vi "Add Address Map Element.vi"(0 "niInstr AXI4-Lite address space v1 FPGA in":refnum<class "niInstr AXI4-Lite Address Space v1 FPGA.lvclass">, 5 "address map element in":T1) -> (4 "niInstr AXI4-Lite address space v1 FPGA out":refnum<class "niInstr AXI4-Lite Address Space v1 FPGA.lvclass">)   [LabVIEW 2015, in "niInstr AXI4-Lite Address Space v1 FPGA.lvclass"]
uses:
  <instrlib>/_niInstr/CLIP Adapters/v1/FPGA/AXI4-Lite/Address Space/niInstr AXI4-Lite Address Space v1 FPGA.lvclass
  <instrlib>/_niInstr/Instruction Framework/v1/FPGA/Typedefs/Address Map Element.ctl
  <instrlib>/_niInstr/CLIP Adapters/v1/FPGA/AXI4-Lite/Address Space/niInstr AXI4-Lite Address Space v1 FPGA.lvclass/niInstr AXI4-Lite Address Space v1 FPGA.ctl
  <instrlib>/_niInstr/Instruction Framework/v1/FPGA/Typedefs/niInstr Instruction Framework v1 FPGA.lvlib
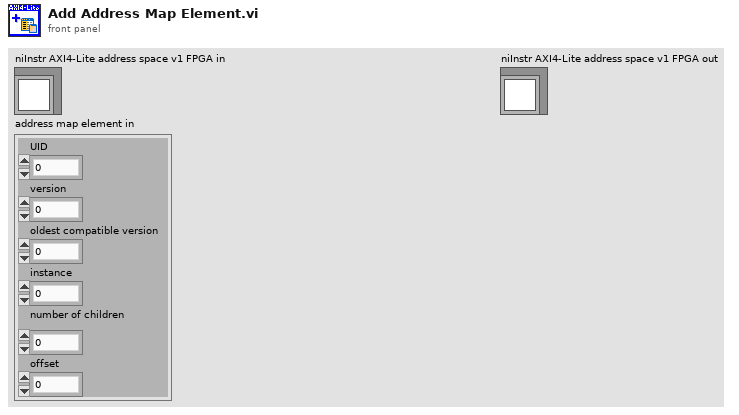
[diagram p1: front panel]
types:
  T1 = typedef "niInstr Instruction Framework v1 FPGA.lvlib/Address Map Element.ctl" = cluster{"UID":u16, "version":u16, "oldest compatible version":u16, "instance":u8, "number of children":u8, "offset":u32}
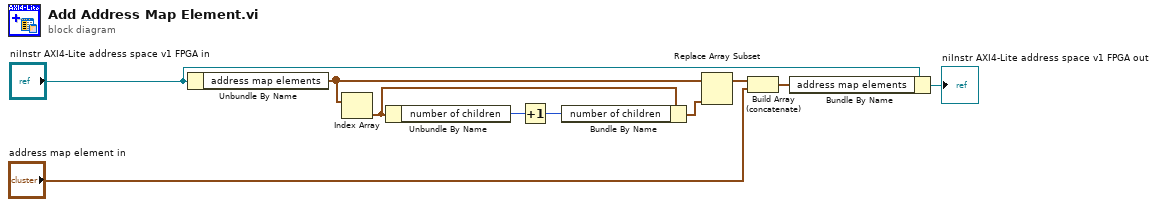
[diagram p0: block diagram]
diagram:
  n1 = Unbundle By Name("niInstr AXI4-Lite address space v1 FPGA in") -> ("address map elements"=w5:T1[])
  n2 = Index Array(array=w5) -> (element=w7:T1)  [unwired: 1 in]
  n3 = Unbundle By Name(w7) -> ("number of children"=w6:u8)
  n4 = Increment(x=w6) -> (x+1=w1:u8)
  n5 = Bundle By Name(cluster=w7, "number of children"=w1) -> (w4:T1)
  n6 = Replace Array Subset(array=w5, new element=w4) -> (w3:T1[])  [unwired: 1 in]
  n7 = Build Array (concatenate)(w3, "address map element in") -> (w2:T1[])
  n8 = Bundle By Name(cluster="niInstr AXI4-Lite address space v1 FPGA in", "address map elements"=w2) -> (→"niInstr AXI4-Lite address space v1 FPGA out":refnum<class "niInstr AXI4-Lite Address Space v1 FPGA.lvclass">)
